vi "Group_ToXML.vi"(8 "error in (no error)":errorcluster, 11 "Group in":refnum<class "Group.lvclass">) -> (0 "error out":errorcluster, 2 "XML String":string, 3 "Group out":refnum<class "Group.lvclass">)   [LabVIEW 2023, in "Group.lvclass"]
doc: "Converts the group definition to XML format and it's subsidiary channels."
uses:
  Group.lvclass
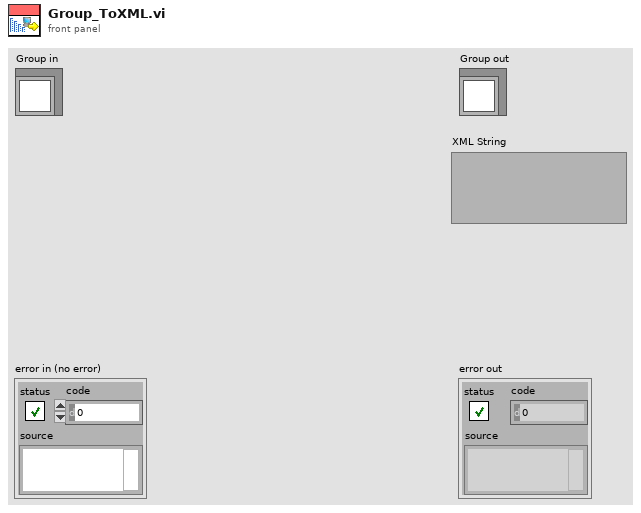
[diagram p1: front panel]
types:
  T1 = typedef "GroupAsCluster.ctl" = cluster{"Name":string, "Channels":T2[], "Meta Data":T4[]}
  T2 = typedef "ChannelAsCluster.ctl" = cluster{"Name":string, "Data Reference":T3, "Wfm?":bool, "Decimation":i32, "Current Value":dbl, "Meta Data":T4[], "WfmPath":string}
  T3 = typedef "Custom Device API.lvlib/Data Reference.ctl" = i32
  T4 = typedef "Meta Data.ctl" = cluster{"Key":string, "Value":string}
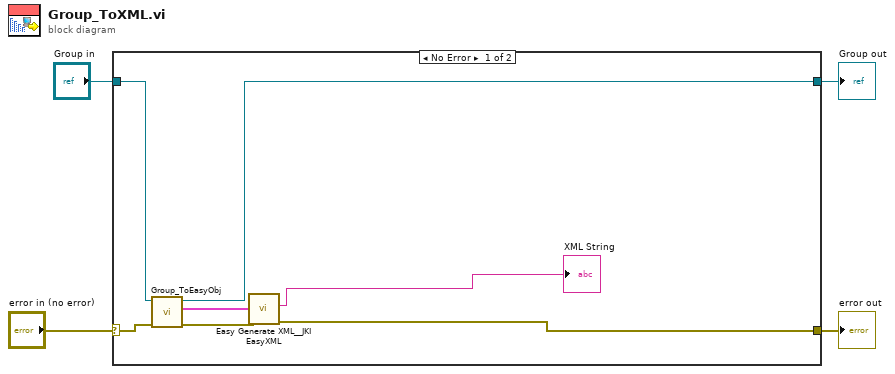
[diagram p0: block diagram]
diagram:
  n1 = case shown="No Error" "error in (no error)" {
    selector: "error in (no error)" -> [w7 w13]
    tunnel: [w10 w13] -> w3
    tunnel: [w5 w12] -> w1
    tunnel: "Group in" -> [w6 w12]
    frame No Error {
      n2 = call-dynamic "Group_ToEasyObj.vi"("error in (no error)"=w7, "Group in"=w6) -> ("error out"=w8:errorcluster, "output cluster"=w9:T1, "Group out"=w5:refnum<class "Group.lvclass">)  [unwired: 7 in]
      n3 = call <vilib>:"Easy Generate XML__JKI EasyXML.vi"("error in (no error)"=w8, "LabVIEW Data"=w9) -> ("error out"=w10:errorcluster, "XML String"=→"XML String":string)  [unwired: 8 in]
    }
    frame Error {
    }
  }
  "error out" <- w3
  "Group out" <- w1
